vi "Gestione misure real time.vi"(11 "lingua":i32) -> ()   [LabVIEW 2019]
uses:
  <vilib>/Utility/miscctls.llb/LVRowAndColumnTypeDef.ctl
  Global percorso impostazioni.vi
  <vilib>/Utility/file.llb/Read Delimited Spreadsheet (string).vi
  <vilib>/Utility/file.llb/Write Delimited Spreadsheet (string).vi
panel:
  in  "TIPO COLLEGAMENTO":u16(ring) items=["GRUPPO ELETTROGENO", "ALTERNATORE", "GENERICO", "MOTORE C.A.", "MOTORE EEX", "MOTORE C.C.", "POMPA", "TRASFORMATORE", "POMPA EEX"]
  in  "set etichetta mono":T1={"Grandezza"="", "Etichetta"="", "conferma"=FALSE, "indice"=0, "posizione"=0, "DIMENSIONE CARATTERE"=30}
  in  "set etichetta tri":T2={"Grandezza"="", "Etichetta"="", "conferma"=FALSE, "indice"=0, "posizione"=0, "DIMENSIONE CARATTERE"=30, "Text color"=16448250}
  in  "aggiungi tri tutti":bool
  in  "aggiungi tri":bool
  in  "salva":bool
  out "String":string
  in  "rimuovi selezionata tri":bool
  in  "Lista grandezze visualizzate":i32(listbox)
  in  "exit":bool
  in  "Lista grandezze":i32(listbox)
  # "clicca e trascina per ordinare\n\nDoppio click sulla riga per modificare etichetta e dimensione carattere"
  # "Nota: trascina per ordinare"
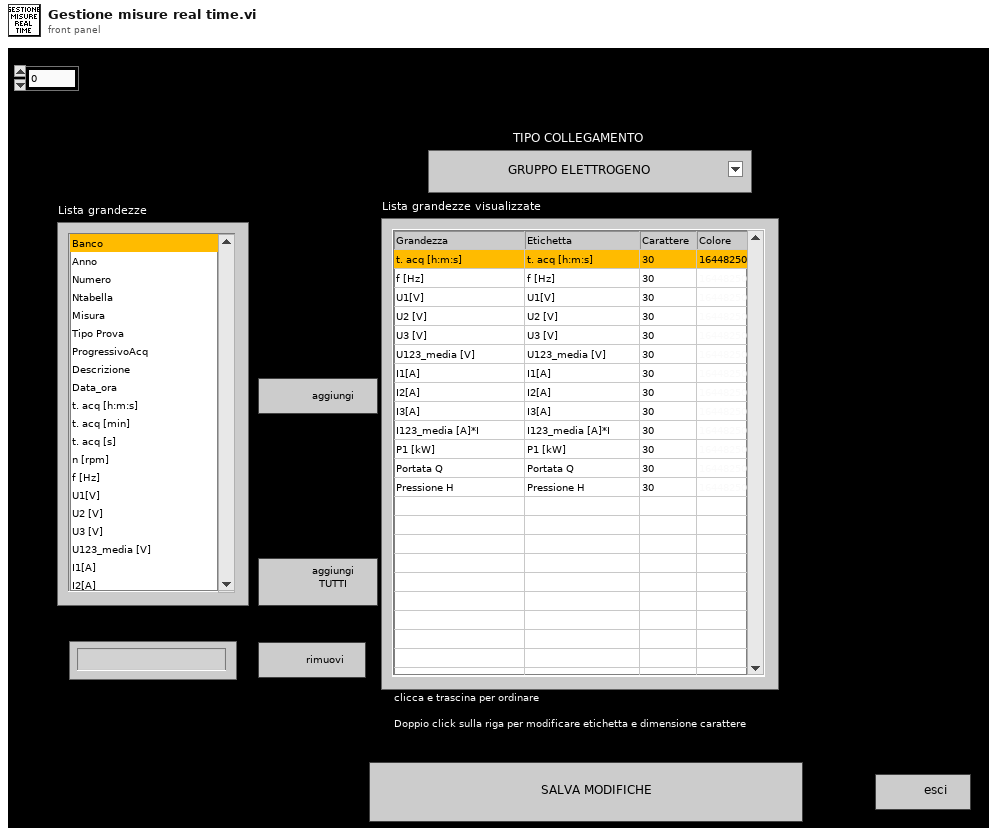
[diagram p1: front panel]
types:
  T1 = cluster{"Grandezza":string, "Etichetta":string, "conferma":bool, "indice":i8, "posizione":i8, "DIMENSIONE CARATTERE":i16}
  T2 = cluster{"Grandezza":string, "Etichetta":string, "conferma":bool, "indice":i8, "posizione":i8, "DIMENSIONE CARATTERE":i16, "Text color":u32}
  T3 = enum8{"Enabled", "Disabled", "Disabled and Grayed Out"}
  T4 = typedef "LVRowAndColumnTypeDef.ctl" = cluster{"Row":i32, "Column":i32}
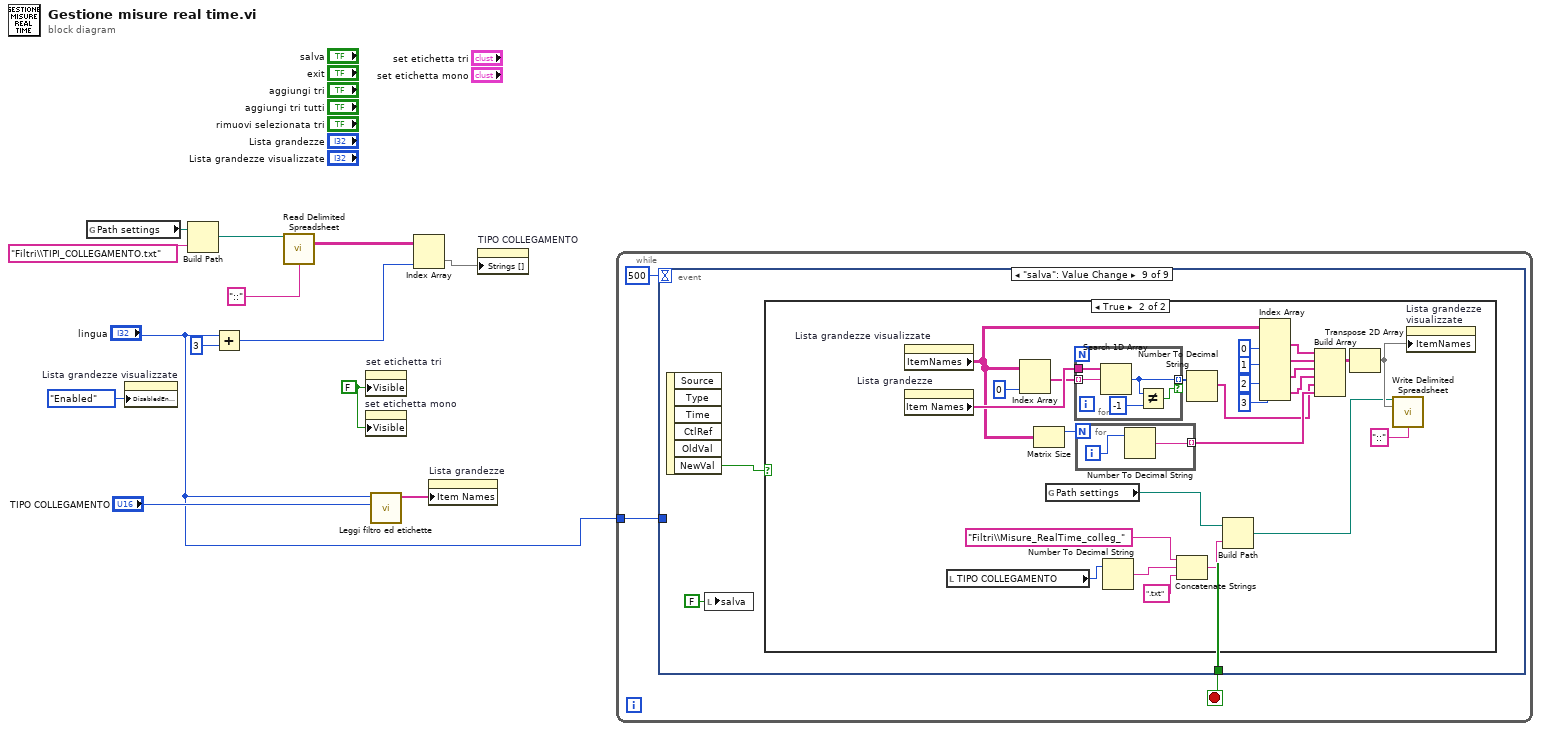
[diagram p0: block diagram]
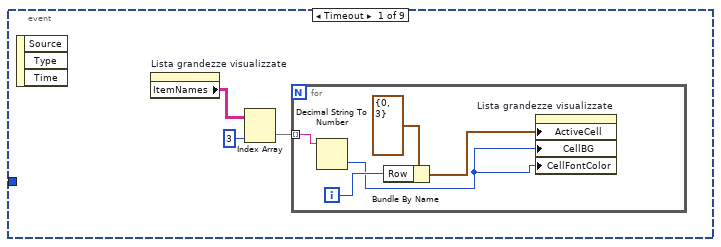
[diagram p2: hidden frame]
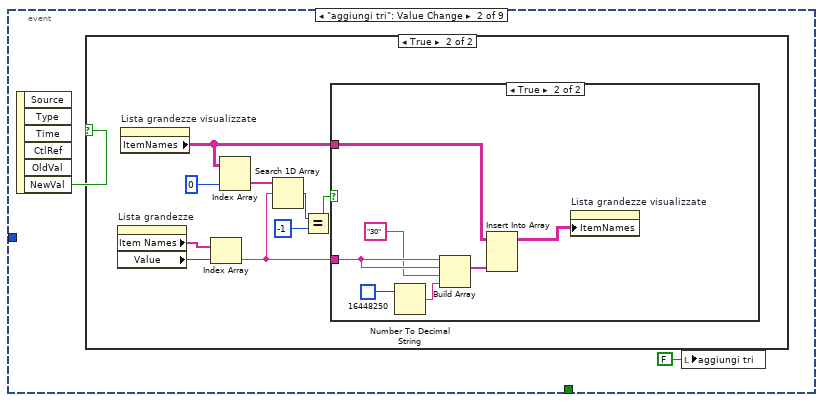
[diagram p3: hidden frame]
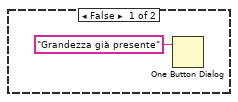
[diagram p5: hidden frame]
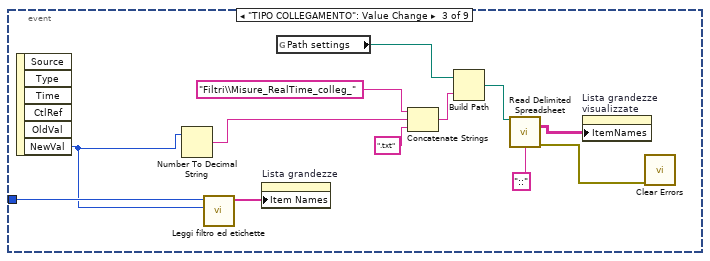
[diagram p6: hidden frame]
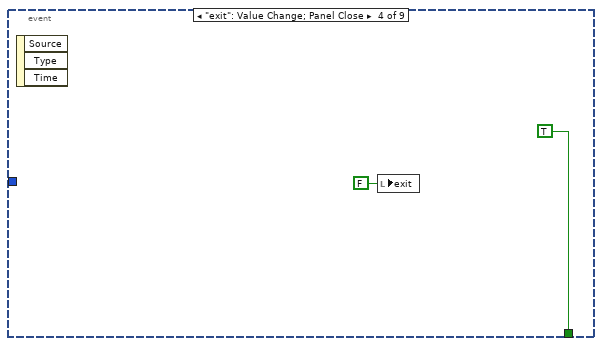
[diagram p7: hidden frame]
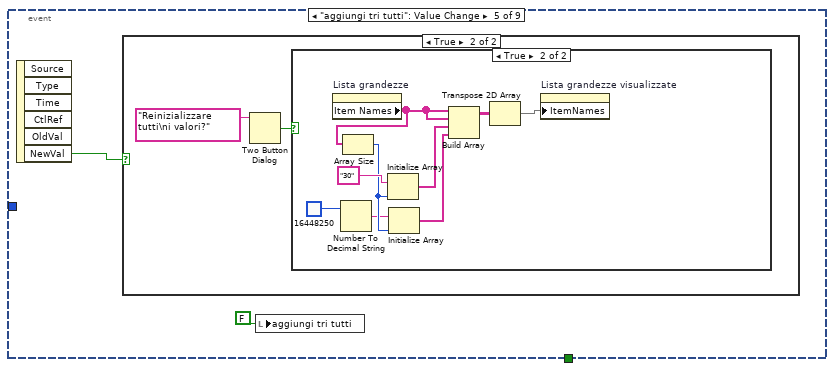
[diagram p8: hidden frame]
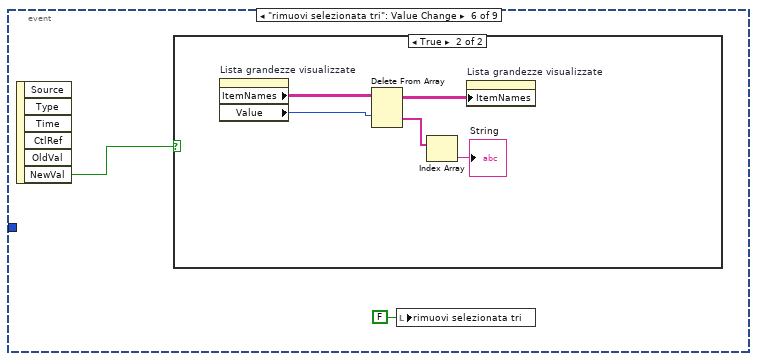
[diagram p11: hidden frame]
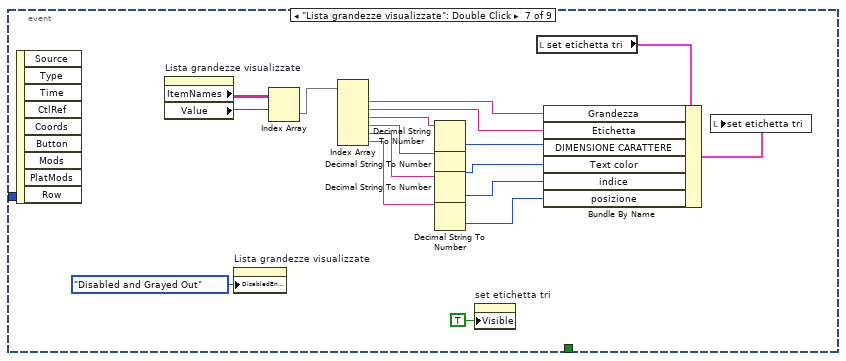
[diagram p13: hidden frame]
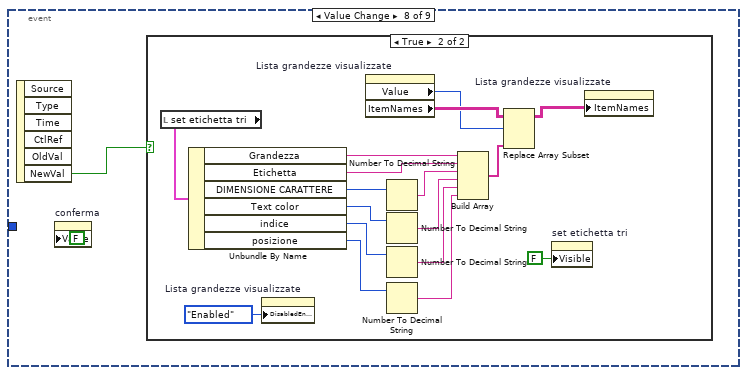
[diagram p14: hidden frame]
diagram:
  w13 = FALSE ("Visible")
  n1 = global read "Global percorso impostazioni.vi" "Path settings"() -> (w10:path)
  n2 = property on="Lista grandezze visualizzate" class="MCListbox (strict)"("DisabledEnum"=T3."Enabled" ("Disabled")) -> ()  [unwired: 2 in, 2 out]
  n3 = Build Path(base path=w10, name or relative path="Filtri\\TIPI_COLLEGAMENTO.txt") -> (appended path=w8:path)
  n4 = Add(x="lingua", y=3) -> (x+y=w5:i32)
  n5 = call-poly <vilib>:"Read Delimited Spreadsheet.vi"("file path (dialog if empty)"=w8, "delimiter (\\t)"="::") -> ("all rows"=w7:string[][])  [unwired: 8 in, 5 out]
  n6 = property on="set etichetta tri" class="Clust (strict)"("Visible"=w13) -> ()  [unwired: 2 in, 2 out]
  n7 = property on="set etichetta mono" class="Clust (strict)"("Visible"=w13) -> ()  [unwired: 2 in, 2 out]
  n8 = call "Leggi filtro ed etichette.vi"("ID COLLEGAMENTO"="TIPO COLLEGAMENTO", "LINGUA"="lingua") -> ("ETICHETTE"=w2:string[])  [unwired: 4 in, 5 out]
  n9 = Index Array(array=w7, index (col)=w5) -> (element=w4:string[])  [unwired: 1 in]
  n10 = property on="Lista grandezze" class="LstBox (strict)"("Item Names"=w2) -> ()  [unwired: 2 in, 2 out]
  n11 = property on="TIPO COLLEGAMENTO" class="Ring (strict)"("Strings []"=w4) -> ()  [unwired: 2 in, 2 out]
  n12 = while {
    tunnel: "lingua" -> [w14]
    stop <- w16 stop-if-true
    n13 = event shown="[8] \"salva\": Value Change" {
      selector: _ -> [_ _ _ _ _ _ _ _ _]
      dyn-events: _ -> [_ _ _ _ _ _ _ _ _]
      timeout: 500 -> [_ _ _ _ _ _ _ _ _]
      tunnel: [_ _ _ TRUE _ _ _ _ _] -> w16
      tunnel: w14 -> [_ _ w54 _ _ _ _ _ _]
      event Timeout {
        n14 = event-data() -> ()  [unwired: 1 in, 3 out]
        n15 = property on="Lista grandezze visualizzate" class="MCListbox (strict)"() -> ("ItemNames"=w19:string[][])  [unwired: 2 in, 2 out]
        n16 = Index Array(array=w19, index (col)=3 ("disabled index (col)")) -> (element=w17:string[])  [unwired: 1 in]
        n17 = for {
          tunnel: w17 -> [w21] mode=indexing
          i -> [w22]
          n18 = Decimal String To Number(string=w21) -> (number=w20:i32)  [unwired: 2 in, 1 out]
          n19 = Bundle By Name(cluster=T4 {"Row"=0, "Column"=3} ("Active Cell:Active Cell"), "Row"=w22) -> (w23:T4)
          n20 = property on="Lista grandezze visualizzate" class="MCListbox (strict)"("ActiveCell"=w23, "CellBG"=w20, "CellFontColor"=w20) -> ()  [unwired: 2 in, 2 out]
        }
      }
      event "aggiungi tri": Value Change {
        n21 = event-data() -> ("NewVal"=w25:bool)  [unwired: 1 in, 5 out]
        n22 = case shown="True" w25 {
          frame False {
          }
          frame True {
            n23 = property on="Lista grandezze" class="LstBox (strict)"() -> ("Item Names"=w35:string[], "Value"=w34:i32)  [unwired: 2 in, 2 out]
            n24 = property on="Lista grandezze visualizzate" class="MCListbox (strict)"() -> ("ItemNames"=w31:string[][])  [unwired: 2 in, 2 out]
            n25 = Index Array(array=w35, index=w34) -> (element=w30:string)
            n26 = Index Array(array=w31, index (col)=0 ("disabled index (col)")) -> (element=w32:string[])  [unwired: 1 in]
            n27 = Search 1D Array(1D array=w32, element=w30) -> (index of element=w28:i32)  [unwired: 1 in]
            n28 = Equal?(x=w28, y=-1) -> (x = y?=w27:bool)
            n29 = case shown="True" w27 {
              tunnel: w31 -> [_ w41]
              tunnel: w30 -> [_ w40]
              frame False {
                n30 = One Button Dialog(message="Grandezza già presente") -> ()  [unwired: 1 in, 1 out]
              }
              frame True {
                n31 = Number To Decimal String(number=u32 16448250 ("Text color")) -> (decimal integer string=w37:string)  [unwired: 1 in]
                n32 = Build Array(w40, w40, "30" ("element"), w37) -> (w42:string[])
                n33 = Insert Into Array(array=w41, new element=w42) -> (w43:string[][])  [unwired: 2 in]
                n34 = property on="Lista grandezze visualizzate" class="MCListbox (strict)"("ItemNames"=w43) -> ()  [unwired: 2 in, 2 out]
              }
            }
          }
        }
        n35 = local write "aggiungi tri"(FALSE ("aggiungi tri")) -> ()
      }
      event "TIPO COLLEGAMENTO": Value Change {
        n36 = event-data() -> ("NewVal"=w51:u16)  [unwired: 1 in, 5 out]
        n37 = Number To Decimal String(number=w51) -> (decimal integer string=w50:string)  [unwired: 1 in]
        n38 = call "Leggi filtro ed etichette.vi"("ID COLLEGAMENTO"=w51, "LINGUA"=w54) -> ("ETICHETTE"=w55:string[])  [unwired: 4 in, 5 out]
        n39 = property on="Lista grandezze" class="LstBox (strict)"("Item Names"=w55) -> ()  [unwired: 2 in, 2 out]
        n40 = global read "Global percorso impostazioni.vi" "Path settings"() -> (w49:path)
        n41 = Concatenate Strings("Filtri\\Misure_RealTime_colleg_" ("name or relative path"), w50, ".txt" ("string")) -> (w48:string)
        n42 = Build Path(base path=w49, name or relative path=w48) -> (appended path=w46:path)
        n43 = call-poly <vilib>:"Read Delimited Spreadsheet.vi"("file path (dialog if empty)"=w46, "delimiter (\\t)"="::" ("delimiter (\\t)")) -> ("all rows"=w45:string[][], "error out"=w44:errorcluster)  [unwired: 8 in, 4 out]
        n44 = property on="Lista grandezze visualizzate" class="MCListbox (strict)"("ItemNames"=w45) -> ()  [unwired: 2 in, 2 out]
        n45 = call <vilib>:"Clear Errors.vi"("error in (no error)"=w44) -> ()  [unwired: 5 in, 2 out]
      }
      event "exit": Value Change; Panel Close {
        n46 = event-data() -> ()  [unwired: 1 in, 3 out]
        n47 = local write "exit"(FALSE ("exit")) -> ()
      }
      event "aggiungi tri tutti": Value Change {
        n48 = event-data() -> ("NewVal"=w59:bool)  [unwired: 1 in, 5 out]
        n49 = case shown="True" w59 {
          frame False {
          }
          frame True {
            n50 = Two Button Dialog(message="Reinizializzare tutti\ni valori?") -> (T button?=w61:bool)  [unwired: 2 in]
            n51 = case shown="True" w61 {
              frame False {
              }
              frame True {
                n52 = property on="Lista grandezze" class="LstBox (strict)"() -> ("Item Names"=w67:string[])  [unwired: 2 in, 2 out]
                n53 = Number To Decimal String(number=u32 16448250 ("Text color")) -> (decimal integer string=w62:string)  [unwired: 1 in]
                n54 = Array Size(array=w67) -> (size(s)=w64:i32)
                n55 = Initialize Array("30", w64) -> (w66:string[])
                n56 = Initialize Array(w62, w64) -> (w65:string[])
                n57 = Build Array(w67, w67, w66, w65) -> (w70:string[][])
                n58 = Transpose 2D Array(2D array=w70) -> (transposed array=w69:string[][])
                n59 = property on="Lista grandezze visualizzate" class="MCListbox (strict)"("ItemNames"=w69) -> ()  [unwired: 2 in, 2 out]
              }
            }
          }
        }
        n60 = local write "aggiungi tri tutti"(FALSE ("aggiungi tri tutti")) -> ()
      }
      event "rimuovi selezionata tri": Value Change {
        n61 = event-data() -> ("NewVal"=w72:bool)  [unwired: 1 in, 5 out]
        n62 = case shown="True" w72 {
          frame False {
          }
          frame True {
            n63 = property on="Lista grandezze visualizzate" class="MCListbox (strict)"() -> ("ItemNames"=w77:string[][], "Value"=w76:i32)  [unwired: 2 in, 2 out]
            n64 = Delete From Array(array=w77, index (row)=w76) -> (deleted portion=w74:string[], array with subset deleted=w75:string[][])  [unwired: 2 in]
            n65 = Index Array(array=w74) -> (element=→"String":string)  [unwired: 1 in]
            n66 = property on="Lista grandezze visualizzate" class="MCListbox (strict)"("ItemNames"=w75) -> ()  [unwired: 2 in, 2 out]
          }
        }
        n67 = local write "rimuovi selezionata tri"(FALSE ("rimuovi selezionata tri")) -> ()
      }
      event "Lista grandezze visualizzate": Double Click {
        n68 = event-data() -> ()  [unwired: 1 in, 9 out]
        n69 = property on="Lista grandezze visualizzate" class="MCListbox (strict)"() -> ("ItemNames"=w94:string[][], "Value"=w93:i32)  [unwired: 2 in, 2 out]
        n70 = property on="Lista grandezze visualizzate" class="MCListbox (strict)"("DisabledEnum"=T3."Disabled and Grayed Out" ("Disabled")) -> ()  [unwired: 2 in, 2 out]
        n71 = Index Array(array=w94, index (row)=w93) -> (element=w92:string[])  [unwired: 1 in]
        n72 = Index Array(array=w92) -> (element #1=w89:string, element #2=w88:string, element #3=w80:string, element #4=w81:string, element #5=w82:string, element #6=w83:string)  [unwired: 6 in]
        n73 = Decimal String To Number(string=w80) -> (number=w79:i32)  [unwired: 2 in, 1 out]
        n74 = Decimal String To Number(string=w81) -> (number=w78:i32)  [unwired: 2 in, 1 out]
        n75 = Decimal String To Number(string=w82) -> (number=w84:i32)  [unwired: 2 in, 1 out]
        n76 = Decimal String To Number(string=w83) -> (number=w85:i32)  [unwired: 2 in, 1 out]
        n77 = property on="set etichetta tri" class="Clust (strict)"("Visible"=TRUE) -> ()  [unwired: 2 in, 2 out]
        n78 = local read "set etichetta tri"() -> (w91:T2)
        n79 = Bundle By Name(cluster=w91, "Grandezza"=w89, "Etichetta"=w88, "DIMENSIONE CARATTERE"=w79, "Text color"=w78, "indice"=w84, "posizione"=w85) -> (w90:T2)
        n80 = local write "set etichetta tri"(w90) -> ()
      }
      event "set etichetta tri.conferma": Value Change {
        n81 = event-data() -> ("NewVal"=w96:bool)  [unwired: 1 in, 5 out]
        n82 = property on="conferma" class="Bool (strict)"("Value"=FALSE) -> ()  [unwired: 2 in, 2 out]
        n83 = case shown="True" w96 {
          frame False {
          }
          frame True {
            n84 = local read "set etichetta tri"() -> (w111:T2)
            n85 = Unbundle By Name(w111) -> ("Grandezza"=w109:string, "Etichetta"=w108:string, "DIMENSIONE CARATTERE"=w102:i16, "Text color"=w98:u32, "indice"=w100:i8, "posizione"=w104:i8)
            n86 = property on="Lista grandezze visualizzate" class="MCListbox (strict)"("DisabledEnum"=T3."Enabled" ("Disabled")) -> ()  [unwired: 2 in, 2 out]
            n87 = property on="Lista grandezze visualizzate" class="MCListbox (strict)"() -> ("Value"=w112:i32, "ItemNames"=w113:string[][])  [unwired: 2 in, 2 out]
            n88 = Number To Decimal String(number=w102) -> (decimal integer string=w101:string)  [unwired: 1 in]
            n89 = Number To Decimal String(number=w98) -> (decimal integer string=w97:string)  [unwired: 1 in]
            n90 = Number To Decimal String(number=w100) -> (decimal integer string=w99:string)  [unwired: 1 in]
            n91 = Number To Decimal String(number=w104) -> (decimal integer string=w103:string)  [unwired: 1 in]
            n92 = Build Array(w109, w108, w101, w97, w99, w103) -> (w107:string[])
            n93 = Replace Array Subset(array=w113, new element=w107, index (row)=w112) -> (w110:string[][])  [unwired: 1 in]
            n94 = property on="set etichetta tri" class="Clust (strict)"("Visible"=FALSE) -> ()  [unwired: 2 in, 2 out]
            n95 = property on="Lista grandezze visualizzate" class="MCListbox (strict)"("ItemNames"=w110) -> ()  [unwired: 2 in, 2 out]
          }
        }
      }
      event "salva": Value Change {
        n96 = event-data() -> ("NewVal"=w115:bool)  [unwired: 1 in, 5 out]
        n97 = local write "salva"(FALSE ("salva")) -> ()
        n98 = case shown="True" w115 {
          frame False {
          }
          frame True {
            n99 = property on="Lista grandezze visualizzate" class="MCListbox (strict)"() -> ("ItemNames"=w131:string[][])  [unwired: 2 in, 2 out]
            n100 = property on="Lista grandezze" class="LstBox (strict)"() -> ("Item Names"=w138:string[])  [unwired: 2 in, 2 out]
            n101 = local read "TIPO COLLEGAMENTO"() -> (w117:u16)
            n102 = Index Array(array=w131, index (col)=0 ("disabled index (col)")) -> (element=w137:string[])  [unwired: 1 in]
            n103 = Matrix Size(0:w131) -> (1:w130:i32)  [unwired: 1 out]
            n104 = global read "Global percorso impostazioni.vi" "Path settings"() -> (w119:path)
            n105 = for {
              tunnel: w138 -> [w145]
              tunnel: w137 -> [w144] mode=indexing
              tunnel: [w148] -> w139 mode=indexing if=w146
              n106 = Search 1D Array(1D array=w145, element=w144) -> (index of element=w148:i32)  [unwired: 1 in]
              n107 = Not Equal?(x=w148, y=-1) -> (x != y?=w146:bool)
            }
            n108 = for {
              N: w130 -> [_]
              tunnel: [w142] -> w125 mode=indexing
              i -> [w143]
              n109 = Number To Decimal String(number=w143) -> (decimal integer string=w142:string)  [unwired: 1 in]
            }
            n110 = Number To Decimal String(number=w117) -> (decimal integer string=w120:string)  [unwired: 1 in]
            n111 = Concatenate Strings("Filtri\\Misure_RealTime_colleg_" ("name or relative path"), w120, ".txt" ("string")) -> (w118:string)
            n112 = Number To Decimal String(number=w139) -> (decimal integer string=w123:string[])  [unwired: 1 in]
            n113 = Build Path(base path=w119, name or relative path=w118) -> (appended path=w116:path)
            n114 = Index Array(array=w131, index (col) #1=0 ("disabled index (col)"), index (col) #2=1 ("index (col)"), index (col) #3=2 ("index (col)"), index (col) #4=3 ("index (col)")) -> (element #1=w133:string[], element #2=w132:string[], element #3=w127:string[], element #4=w124:string[])  [unwired: 4 in]
            n115 = Build Array(w133, w132, w127, w124, w123, w125) -> (w141:string[][])
            n116 = Transpose 2D Array(2D array=w141) -> (transposed array=w129:string[][])
            n117 = call-poly <vilib>:"Write Delimited Spreadsheet.vi"("file path (dialog if empty)"=w116, "2D data"=w129, "delimiter (\\t)"="::" ("delimiter (\\t)")) -> ()  [unwired: 11 in, 2 out]
            n118 = property on="Lista grandezze visualizzate" class="MCListbox (strict)"("ItemNames"=w129) -> ()  [unwired: 2 in, 2 out]
          }
        }
      }
    }
  }
